vi "Add single ROI overlay.vi"(6 "Abs. index of selected Z-plane (unity-based)":i32, 7 "Number of Z-planes":i32, 8 "ROI Properties":T1 {"Z stop" format="%#_6f"; "Z start" format="%#_6f"; "ROI group ID" format="%#_6f"; "Laser Power (%)" format="%#_6f"; "Zoom" format="%#_6f"; "Frame Size" format="%#_6f"; "Number of lines" format="%#_6f"; "Composite ID" format="%#_6f"; "Angle (deg)" format="%#_6f"; "ROI Time (ns)" format="%#_6f"; "ROI ID" format="%#_6f"; "Pixels in ROI" format="%#_6f"; "ROI index" format="%#_6f"; "Y stop" format="%#_6f"; "X stop" format="%#_6f"; "X start" format="%#_6f"; "Y start" format="%#_6f"}, 9 "Z code":u8, 10 "Image2":T2, 11 "Image1":T2) -> (0 "Error out":errorcluster, 2 "Image2 Out":T2, 3 "Image1 Out":T2)   [LabVIEW 2017]
uses:
  <vilib>/vision/Image Controls.llb/IMAQ Image.ctl
  Typedefs/ROI parameters data type.ctl
panel:
  in  "Volume Colour":u32(colorbox)=27903
  in  "Rectangular text Colour":u32(colorbox)=6618880
  in  "Rectangular line Colour":u32(colorbox)=56063
  in  "POI text Colour":u32(colorbox)=6618880
  in  "Miniscan text colour":u32(colorbox)=6618880
  in  "POI line Colour":u32(colorbox)=16711680
  in  "Miniscan line colour":u32(colorbox)=16682774
  in  "Text Colour":u32(colorbox)=13882323
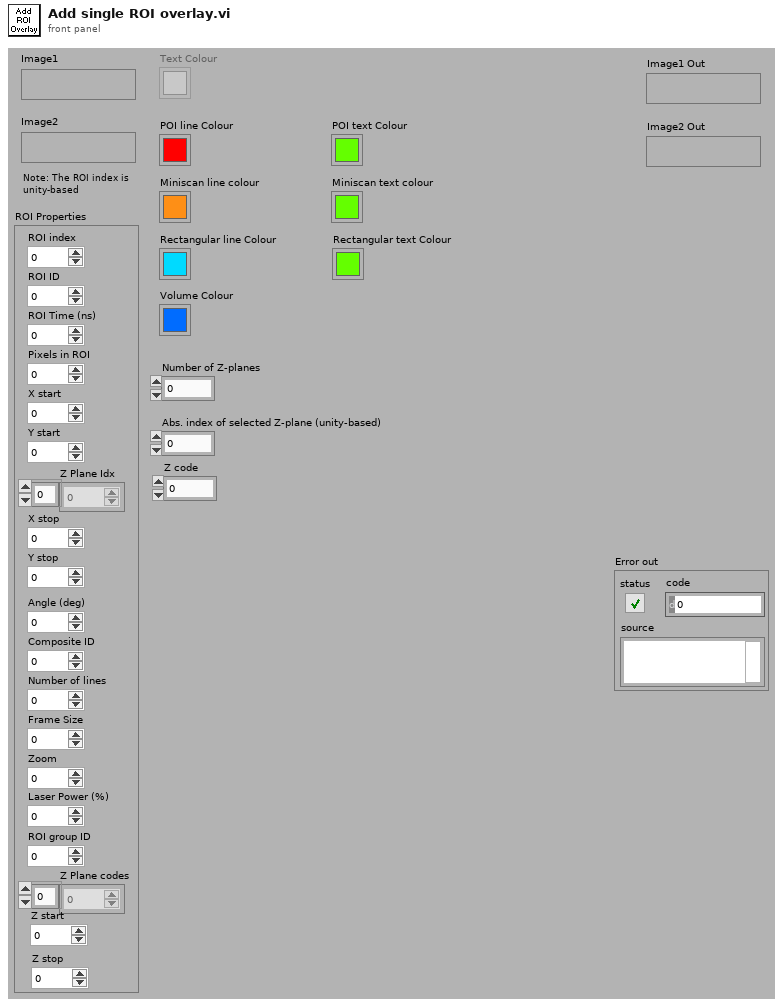
[diagram p1: front panel]
types:
  T1 = typedef "ROI parameters data type.ctl" = cluster{"ROI index":dbl, "ROI ID":dbl, "ROI Time (ns)":dbl, "Pixels in ROI":dbl, "X start":dbl, "Y start":dbl, "X stop":dbl, "Y stop":dbl, "Angle (deg)":dbl, "Composite ID":dbl, "Number of lines":dbl, "Frame Size":dbl, "Zoom":dbl, "Laser Power (%)":dbl, "ROI group ID":dbl, "Z Plane Idx":i32[], "Z Plane codes":u8[], "Z start":dbl, "Z stop":dbl}
  T2 = typedef "IMAQ Image.ctl" = refnum<image>
  T3 = cluster{"Left":i32, "Top":i32, "Right":i32, "Bottom":i32}
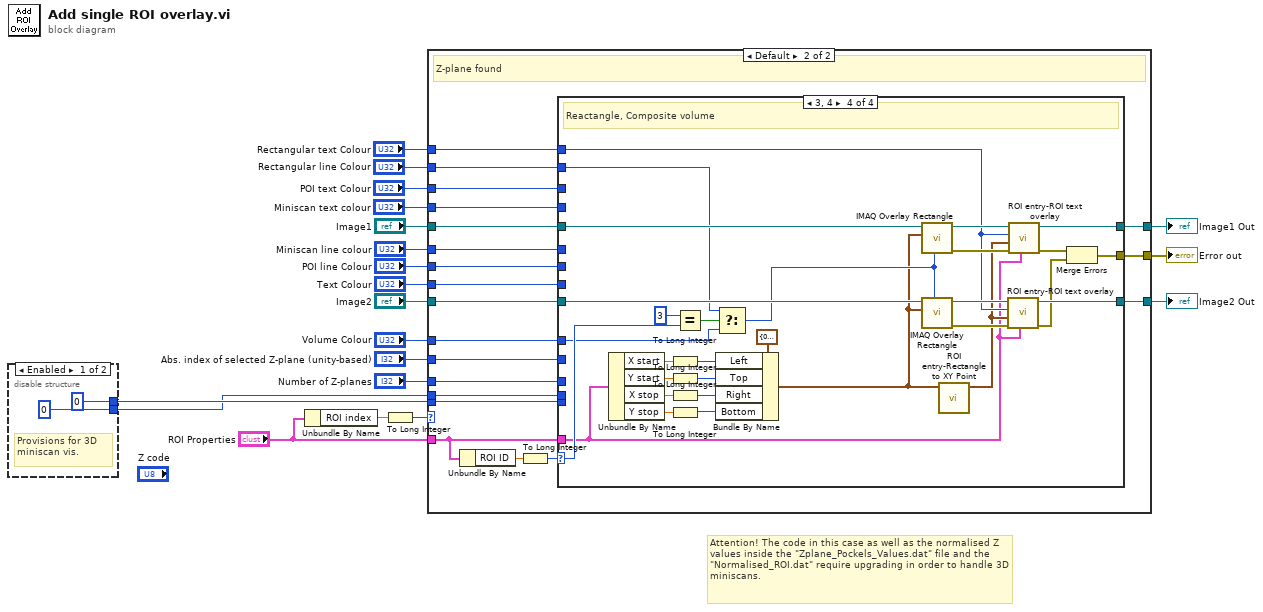
[diagram p0: block diagram]
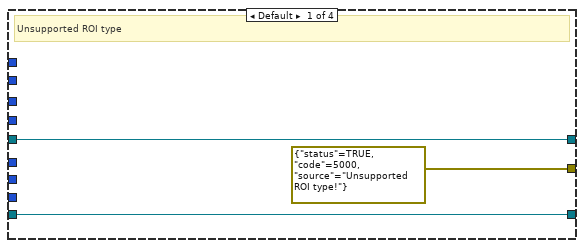
[diagram p4: hidden frame]
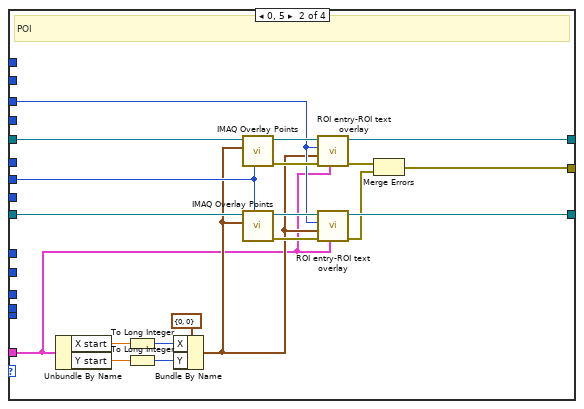
[diagram p5: hidden frame]
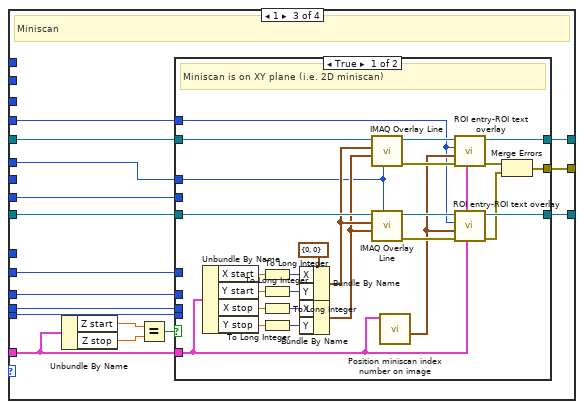
[diagram p6: hidden frame]
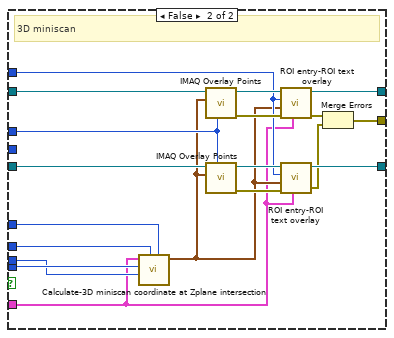
[diagram p7: hidden frame]
diagram:
  # "Attention! The code in this case as well as the normalised Z values inside the \"Zplane_Pockels_Values.dat\" file and the \"Normalised_ROI.dat\" require upgrading in order to handle 3D miniscans."
  n1 = disable-structure "Diagram Disable Structure" shown="Enabled" {
    disable-tunnel: [0 ("Number of intersected Zplanes") _] -> w11
    disable-tunnel: [0 ("Number of intersected Zplanes") _] -> w10
    frame Enabled {
      # "Provisions for 3D miniscan vis."
    }
    frame Disabled {
    }
  }
  n2 = Unbundle By Name("ROI Properties") -> ("ROI index"=w16:dbl)
  n3 = To Long Integer(number=w16) -> (32bit integer=w1:i32)
  n4 = case shown="Default" w1 {
    tunnel: "Image1" -> [w24 w44]
    tunnel: "Image2" -> [w23 w43]
    tunnel: [w24 w42] -> w19
    tunnel: [w23 w41] -> w18
    tunnel: "ROI Properties" -> [_ w39]
    tunnel: "Text Colour" -> [_ w38]
    tunnel: "Number of Z-planes" -> [_ w36]
    tunnel: "Abs. index of selected Z-plane (unity-based)" -> [_ w37]
    tunnel: w11 -> [_ w35]
    tunnel: w10 -> [_ w34]
    tunnel: "POI line Colour" -> [_ w33]
    tunnel: "Miniscan line colour" -> [_ w32]
    tunnel: "Miniscan text colour" -> [_ w31]
    tunnel: "POI text Colour" -> [_ w30]
    tunnel: [_ w29] -> w5
    tunnel: "Rectangular text Colour" -> [_ w28]
    tunnel: "Rectangular line Colour" -> [_ w27]
    tunnel: "Volume Colour" -> [_ w26]
    frame -1 {
      # "Z-plane not found"
    }
    frame Default {
      # "Z-plane found"
      n5 = Unbundle By Name(w39) -> ("ROI ID"=w40:dbl)
      n6 = To Long Integer(number=w40) -> (32bit integer=w25:i32)
      n7 = case shown="3, 4" w25 {
        selector: w25 -> [_ _ _ w146]
        tunnel: w44 -> [w47 w63 w83 w158]
        tunnel: w43 -> [w46 w62 w82 w157]
        tunnel: [w47 w61 w81 w139] -> w42
        tunnel: [w46 w60 w80 w135] -> w41
        tunnel: w39 -> [_ w48 w68 w129]
        tunnel: w38 -> [_ _ w76 _]
        tunnel: w37 -> [_ _ w75 _]
        tunnel: w36 -> [_ _ w74 _]
        tunnel: w35 -> [_ _ w73 _]
        tunnel: w34 -> [_ _ w72 _]
        tunnel: w33 -> [_ w53 _ _]
        tunnel: w32 -> [_ _ w71 _]
        tunnel: w31 -> [_ _ w70 _]
        tunnel: w30 -> [_ w54 _ _]
        tunnel: [errorcluster {"status"=TRUE, "code"=5000, "source"="Unsupported ROI type!"} ("error IO") w50 w69 w156] -> w29
        tunnel: w28 -> [_ _ _ w134]
        tunnel: w27 -> [_ _ _ w142]
        tunnel: w26 -> [_ _ _ w143]
        frame Default {
          # "Unsupported ROI type"
        }
        frame 0, 5 {
          # "POI"
          n8 = Unbundle By Name(w48) -> ("X start"=w58:dbl, "Y start"=w57:dbl)
          n9 = To Long Integer(number=w58) -> (32bit integer=w56:i32)
          n10 = To Long Integer(number=w57) -> (32bit integer=w55:i32)
          n11 = Bundle By Name(cluster=cluster{"X":i32, "Y":i32} {"X"=0, "Y"=0} ("Point"), "X"=w56, "Y"=w55) -> (w49:cluster{"X":i32, "Y":i32})
          n12 = call "IMAQ Overlay Points"("Color"=w53, "Point"=w49, "Image"=w63) -> ("error out"=w64:errorcluster, "Image Out"=w65:T2)  [unwired: 7 in]
          n13 = call "IMAQ Overlay Points"("Color"=w53, "Point"=w49, "Image"=w62) -> ("error out"=w67:errorcluster, "Image Out"=w66:T2)  [unwired: 7 in]
          n14 = call "ROI entry-ROI text overlay.vi"("ROI properties"=w48, "Error in (no error)"=w64, "Point"=w49, "Rect. text colour"=w54, "Refnum in"=w65) -> ("error out"=w52:errorcluster, "Refnum out"=w61:T2)  [unwired: 5 in]
          n15 = call "ROI entry-ROI text overlay.vi"("ROI properties"=w48, "Error in (no error)"=w67, "Point"=w49, "Rect. text colour"=w54, "Refnum in"=w66) -> ("error out"=w51:errorcluster, "Refnum out"=w60:T2)  [unwired: 5 in]
          n16 = Merge Errors(w52, w51) -> (w50:errorcluster)
        }
        frame 1 {
          # "Miniscan"
          n17 = Unbundle By Name(w68) -> ("Z start"=w79:dbl, "Z stop"=w78:dbl)
          n18 = Equal?(x=w79, y=w78) -> (x = y?=w77:bool)
          n19 = case shown="True" w77 {
            tunnel: w83 -> [w105 w124]
            tunnel: w82 -> [w104 w123]
            tunnel: [w103 w122] -> w81
            tunnel: [w102 w121] -> w80
            tunnel: w68 -> [w84 w110]
            tunnel: w71 -> [w89 w115]
            tunnel: w76 -> [_ _]
            tunnel: w75 -> [_ w120]
            tunnel: w74 -> [_ w119]
            tunnel: w73 -> [_ w118]
            tunnel: w72 -> [_ w117]
            tunnel: w70 -> [w88 w116]
            tunnel: [w86 w112] -> w69
            frame True {
              w100 = cluster{"X":i32, "Y":i32} {"X"=0, "Y"=0} ("Point")
              # "Miniscan is on XY plane (i.e. 2D miniscan)"
              n20 = Unbundle By Name(w84) -> ("X start"=w90:dbl, "Y start"=w91:dbl, "X stop"=w92:dbl, "Y stop"=w93:dbl)
              n21 = To Long Integer(number=w90) -> (32bit integer=w98:i32)
              n22 = To Long Integer(number=w91) -> (32bit integer=w96:i32)
              n23 = To Long Integer(number=w92) -> (32bit integer=w95:i32)
              n24 = To Long Integer(number=w93) -> (32bit integer=w97:i32)
              n25 = Bundle By Name(cluster=w100, "X"=w98, "Y"=w96) -> (w101:cluster{"X":i32, "Y":i32})
              n26 = Bundle By Name(cluster=w100, "X"=w95, "Y"=w97) -> (w99:cluster{"X":i32, "Y":i32})
              n27 = call "IMAQ Overlay Line"("Color"=w89, "End Point"=w99, "Start Point"=w101, "Image"=w105) -> ("error out"=w106:errorcluster, "Image Out"=w107:T2)  [unwired: 6 in]
              n28 = call "IMAQ Overlay Line"("Color"=w89, "End Point"=w99, "Start Point"=w101, "Image"=w104) -> ("error out"=w109:errorcluster, "Image Out"=w108:T2)  [unwired: 6 in]
              n29 = call "Position miniscan index number on image.vi"("X-Y-Z coordinates"=w84) -> ("X-Y coordinates at miniscan middle point"=w94:cluster{"X":i32, "Y":i32})  [unwired: 10 in]
              n30 = call "ROI entry-ROI text overlay.vi"("ROI properties"=w84, "Error in (no error)"=w106, "Point"=w94, "Rect. text colour"=w88, "Refnum in"=w107) -> ("error out"=w87:errorcluster, "Refnum out"=w103:T2)  [unwired: 5 in]
              n31 = call "ROI entry-ROI text overlay.vi"("ROI properties"=w84, "Error in (no error)"=w109, "Point"=w94, "Rect. text colour"=w88, "Refnum in"=w108) -> ("error out"=w85:errorcluster, "Refnum out"=w102:T2)  [unwired: 5 in]
              n32 = Merge Errors(w87, w85) -> (w86:errorcluster)
            }
            frame False {
              # "3D miniscan"
              n33 = call "Calculate-3D miniscan coordinate at Zplane intersection.vi"("Abs. index of selected Z-plane (unity-based)"=w120, "Number of Z-planes"=w119, "Relative index of selected Z-plane (unity-based)"=w117, "Number of intersected Zplanes"=w118, "input cluster"=w110) -> ("£D miniscan Z-plane intersection coordinates"=w111:cluster{"X":i32, "Y":i32})  [unwired: 6 in]
              n34 = call "IMAQ Overlay Points"("Color"=w115, "Point"=w111, "Image"=w124) -> ("error out"=w125:errorcluster, "Image Out"=w126:T2)  [unwired: 7 in]
              n35 = call "IMAQ Overlay Points"("Color"=w115, "Point"=w111, "Image"=w123) -> ("error out"=w128:errorcluster, "Image Out"=w127:T2)  [unwired: 7 in]
              n36 = call "ROI entry-ROI text overlay.vi"("ROI properties"=w110, "Error in (no error)"=w125, "Point"=w111, "Rect. text colour"=w116, "Refnum in"=w126) -> ("error out"=w114:errorcluster, "Refnum out"=w122:T2)  [unwired: 5 in]
              n37 = call "ROI entry-ROI text overlay.vi"("ROI properties"=w110, "Error in (no error)"=w128, "Point"=w111, "Rect. text colour"=w116, "Refnum in"=w127) -> ("error out"=w113:errorcluster, "Refnum out"=w121:T2)  [unwired: 5 in]
              n38 = Merge Errors(w114, w113) -> (w112:errorcluster)
            }
          }
        }
        frame 3, 4 {
          # "Reactangle, Composite volume"
          n39 = Unbundle By Name(w129) -> ("X start"=w149:dbl, "Y start"=w153:dbl, "X stop"=w154:dbl, "Y stop"=w155:dbl)
          n40 = To Long Integer(number=w149) -> (32bit integer=w148:i32)
          n41 = To Long Integer(number=w153) -> (32bit integer=w147:i32)
          n42 = To Long Integer(number=w154) -> (32bit integer=w151:i32)
          n43 = To Long Integer(number=w155) -> (32bit integer=w150:i32)
          n44 = Equal?(x=3, y=w146) -> (x = y?=w144:bool)
          n45 = Bundle By Name(cluster=T3 {"Left"=0, "Top"=0, "Right"=0, "Bottom"=0} ("Rectangle"), "Left"=w148, "Top"=w147, "Right"=w151, "Bottom"=w150) -> (w131:T3)
          n46 = Select(t=w142, s=w144, f=w143) -> (s? t:f=w141:u32)
          n47 = call "IMAQ Overlay Rectangle"("Color"=w141, "Rectangle"=w131, "Image"=w158) -> ("error out"=w137:errorcluster, "Image Out"=w140:T2)  [unwired: 7 in]
          n48 = call "IMAQ Overlay Rectangle"("Color"=w141, "Rectangle"=w131, "Image"=w157) -> ("error out"=w132:errorcluster, "Image Out"=w136:T2)  [unwired: 7 in]
          n49 = call "ROI entry-Rectangle to XY Point.vi"("Rectangle"=w131) -> ("XY"=w130:cluster{"X":i32, "Y":i32})  [unwired: 10 in]
          n50 = call "ROI entry-ROI text overlay.vi"("ROI properties"=w129, "Error in (no error)"=w132, "Point"=w130, "Rect. text colour"=w134, "Refnum in"=w136) -> ("error out"=w133:errorcluster, "Refnum out"=w135:T2)  [unwired: 5 in]
          n51 = call "ROI entry-ROI text overlay.vi"("ROI properties"=w129, "Error in (no error)"=w137, "Point"=w130, "Rect. text colour"=w134, "Refnum in"=w140) -> ("error out"=w138:errorcluster, "Refnum out"=w139:T2)  [unwired: 5 in]
          n52 = Merge Errors(w138, w133) -> (w156:errorcluster)
        }
      }
    }
  }
  "Image1 Out" <- w19
  "Image2 Out" <- w18
  "Error out" <- w5
